vi "feladat_3.vi"() -> ()   [LabVIEW 2021]
uses:
  <vilib>/Analysis/NI_AALPro.lvlib
panel:
  out "Histogram":i32[](array[numeric])
  out "Histogram Graph":T1(graph)
  in  "Gomb":bool
  out "Boolean":bool
  out "sum":i64
  out "Array":i64[](array[numeric])
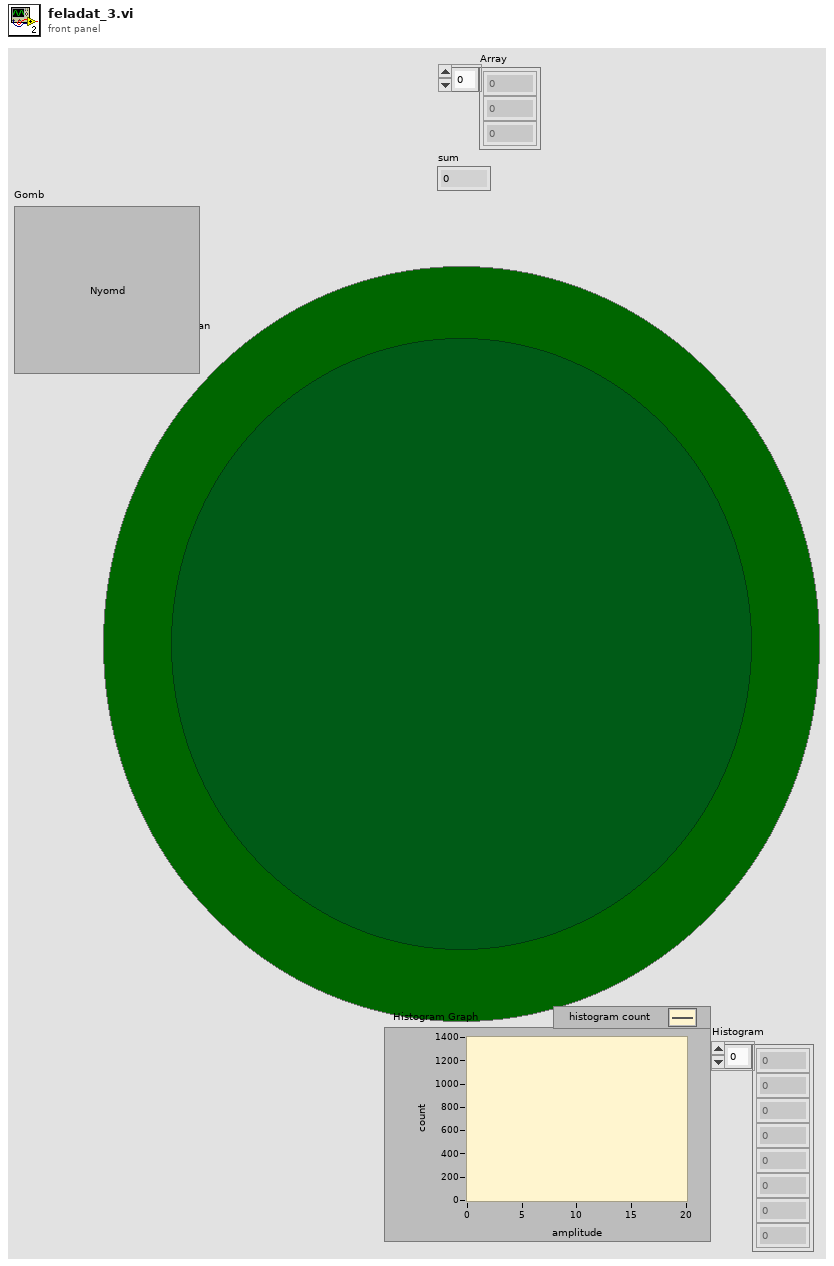
[diagram p1: front panel]
types:
  T1 = cluster{"X Values":dbl[], "Histogram: h(x)":i32[]}
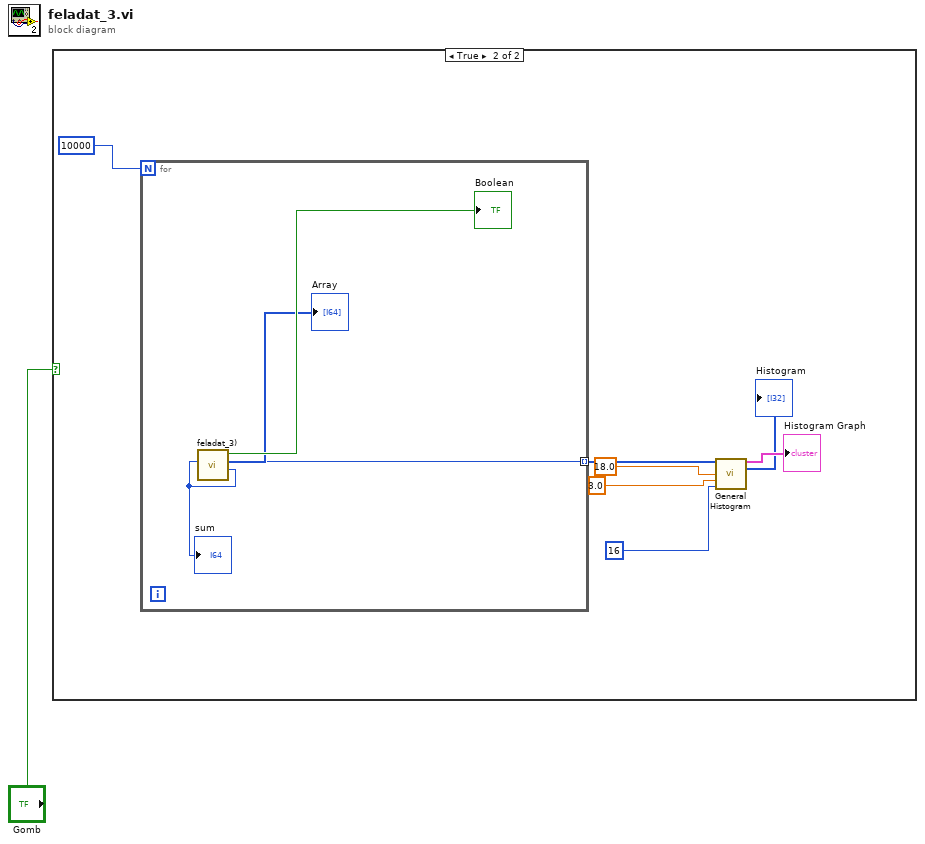
[diagram p0: block diagram]
diagram:
  n1 = case shown="True" "Gomb" {
    frame False {
    }
    frame True {
      n2 = for {
        N: 10000 -> [_]
        tunnel: [w9] -> w3 mode=indexing
        n3 = call "feladat_3).vi"() -> ("number"=w9:i64, "Array"=→"Array":i64[], "Boolean"=→"Boolean":bool)  [unwired: 9 in]
        "sum" <- w9
      }
      n4 = call <vilib>:"General Histogram.vi"("X"=w3, "max"=18.0, "min"=3.0, "# bins"=16) -> ("Histogram Graph"=→"Histogram Graph":T1, "Histogram"=→"Histogram":i32[])  [unwired: 7 in, 3 out]
    }
  }
